vi "connectErrorWires.vi"(8 "error in (no error)":errorcluster, 11 "PolymorphicInstance in":refnum<class "PolymorphicInstance.lvclass">) -> (0 "error out":errorcluster, 3 "PolymorphicInstance out":refnum<class "PolymorphicInstance.lvclass">)   [LabVIEW 2012, in "PolymorphicInstance.lvclass"]
uses:
  PolymorphicInstance.lvclass
  PolymorphicInstance.lvclass/PolymorphicInstance.ctl
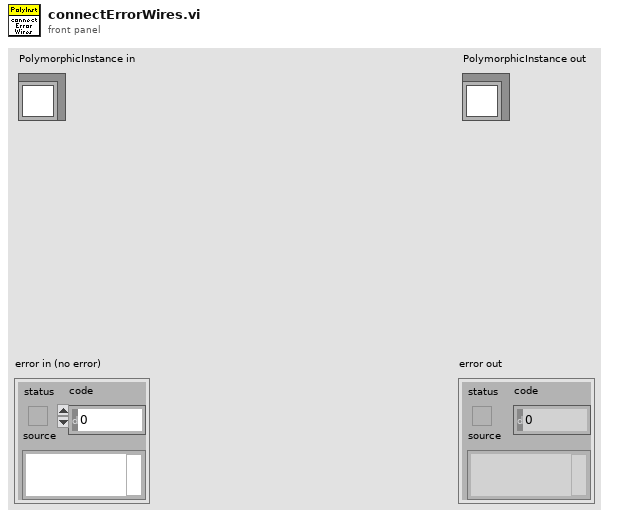
[diagram p1: front panel]
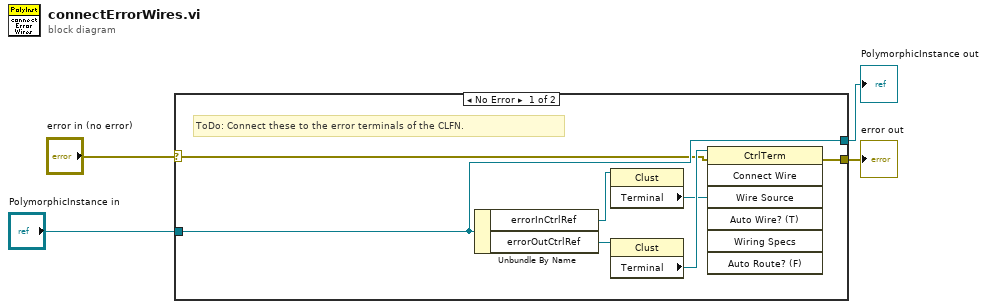
[diagram p0: block diagram]
diagram:
  n1 = case shown="No Error" "error in (no error)" {
    selector: "error in (no error)" -> [w6 w13]
    tunnel: [w5 w13] -> w3
    tunnel: [w9 w12] -> w1
    tunnel: "PolymorphicInstance in" -> [w9 w12]
    frame No Error {
      # "ToDo: Connect these to the error terminals of the CLFN."
      n2 = Unbundle By Name(w9) -> ("errorInCtrlRef"=w7:refnum<vi>, "errorOutCtrlRef"=w8:refnum<vi>)
      n3 = property class="Clust"(reference=w7) -> ("Terminal"=w10:refnum<vi>)  [unwired: 1 in, 2 out]
      n4 = property class="Clust"(reference=w8) -> ("Terminal"=w11:refnum<vi>)  [unwired: 1 in, 2 out]
      n5 = invoke class="CtrlTerm" method="Connect Wire"(reference=w11, error in=w6, "Wire Source"=w10) -> (error out=w5:errorcluster)  [unwired: 4 in, 6 out]
    }
    frame Error {
    }
  }
  "error out" <- w3
  "PolymorphicInstance out" <- w1
